vi "Test Counter Driven Output.vi"(8 "error in":errorcluster, 10 "TestCase in":refnum<class "Scan Engine Scripting API Modules.lvclass">, 11 "module test in":refnum<class "Module Test.lvclass">) -> (0 "error out":errorcluster, 2 "TestCase out":refnum<class "Scan Engine Scripting API Modules.lvclass">, 3 "module test out":refnum<class "Module Test.lvclass">)   [LabVIEW 2017, in "Module Test.lvclass"]
uses:
  Module Test.lvclass
  Scan Engine Scripting API Modules.lvclass
  C:/Program Files (x86)/National Instruments/LabVIEW 2017/vi.lib/addons/_JKI Toolkits/VI Tester/TestCase.llb/TestCase.lvclass
  Scripting/Modules/Mode Classes/Controls/counter driven output channel settings.ctl
  Scripting/Modules/Channel Classes/Counter Driven Output Channel/Counter Driven State.ctl
  Scripting/Modules/Mode Classes/Counter Driven Output Mode/Drive from Slot.ctl
  Module Test.lvclass/Module Test.ctl
  Scripting/Modules/Channel Classes/Counter Driven Output Channel/Counter Driven Output Channel.lvclass
  Scripting/Scan Engine Scripting.lvlib
  Scripting/Modules/Mode Classes/Counter Driven Output Mode/Counter Driven Output Mode.lvclass
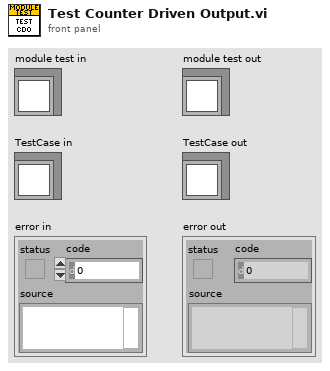
[diagram p1: front panel]
types:
  T1 = typedef "Scan Engine Scripting.lvlib/Counter Driven Output Mode.lvclass/Drive from Slot.ctl" = enum16{"Slot 1", "Slot 2", "Slot 3", "Slot 4", "Slot 5", "Slot 6", "Slot 7", "Slot 8"}
  T2 = typedef "Scan Engine Scripting.lvlib/counter driven output channel settings.ctl" = cluster{"name":string, "default value":bool, "counter driven state":T3}
  T3 = typedef "Scan Engine Scripting.lvlib/Counter Driven Output Channel.lvclass/Counter Driven State.ctl" = enum16{"Disabled", "Enabled"}
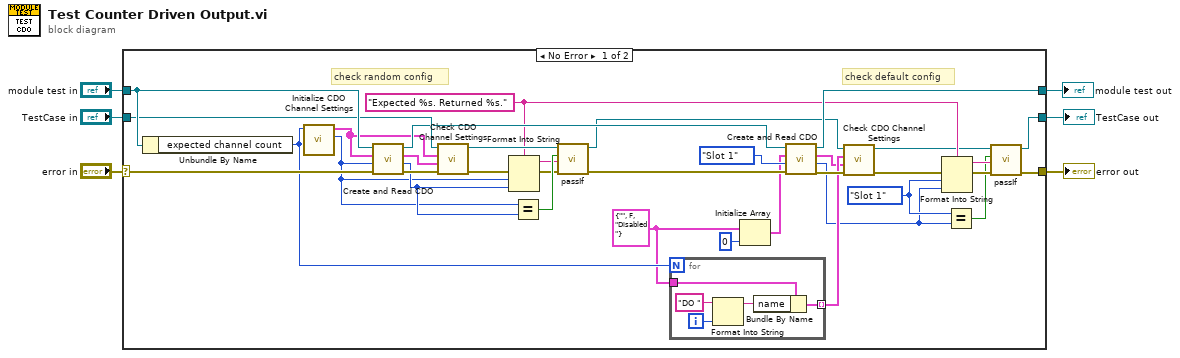
[diagram p0: block diagram]
diagram:
  n1 = case shown="No Error" "error in" {
    selector: "error in" -> [w41 w49]
    tunnel: [w24 w49] -> w5
    tunnel: [w30 w48] -> w3
    tunnel: "module test in" -> [w40 w48]
    tunnel: "TestCase in" -> [w38 w47]
    tunnel: [w25 w47] -> w1
    frame No Error {
      w23 = Drive_from_Slot."Slot 1" ("drive from slot")
      w15 = T2 {"name"="", "default value"=FALSE, "counter driven state"=enum."Disabled"} ("channel settings in")
      w26 = "Expected %s. Returned %s." ("format string")
      # "check default config"
      # "check random config"
      n2 = Unbundle By Name(w40) -> ("expected channel count"=w17:i32)
      n3 = call "Initialize CDO Channel Settings.vi"("array size"=w17) -> ("drive from slot"=w9:T1, "channel settings"=w7:T2[])  [unwired: 9 in]
      n4 = call-dynamic "Create and Read CDO.vi"("error in"=w41, "drive from slot in"=w9, "channel settings in"=w7, "Module Test in"=w40) -> ("error out"=w39:errorcluster, "drive from slot out"=w10:T1, "channel settings out"=w8:T2[], "Module Test out"=w31:refnum<class "Module Test.lvclass">)  [unwired: 4 in]
      n5 = call "Check CDO Channel Settings.vi"("error in"=w39, "read channel settings"=w8, "initial channel settings"=w7, "TestCase in"=w38) -> ("error out"=w34:errorcluster, "TestCase out"=w35:refnum<class "Scan Engine Scripting API Modules.lvclass">)  [unwired: 6 in]
      n6 = Format Into String(format string=w26, error in=w34, w9, w10) -> (resulting string=w33:string, error out=w36:errorcluster)  [unwired: 1 in]
      n7 = Equal?(x=w9, y=w10) -> (x = y?=w37:bool)
      n8 = call-dynamic "passIf.vi"("error in (no error)"=w36, "message (\"\")"=w33, "pass"=w37, "TestCase in"=w35) -> ("error out"=w32:errorcluster, "TestCase out"=w22:refnum<class "Scan Engine Scripting API Modules.lvclass">)  [unwired: 6 in]
      n9 = for {
        N: w17 -> [_]
        tunnel: [w43] -> w18 mode=indexing
        tunnel: w15 -> [w42]
        i -> [w46]
        n10 = Format Into String(initial string="DO ", w46) -> (resulting string=w44:string)  [unwired: 2 in, 1 out]
        n11 = Bundle By Name(cluster=w42, "name"=w44) -> (w43:T2)
      }
      n12 = Initialize Array(w15, 0 ("dimension size")) -> (w13:T2[])
      n13 = call-dynamic "Create and Read CDO.vi"("error in"=w32, "drive from slot in"=Drive_from_Slot."Slot 1", "channel settings in"=w13, "Module Test in"=w31) -> ("error out"=w20:errorcluster, "drive from slot out"=w12:T1, "channel settings out"=w11:T2[], "Module Test out"=w30:refnum<class "Module Test.lvclass">)  [unwired: 4 in]
      n14 = call "Check CDO Channel Settings.vi"("error in"=w20, "read channel settings"=w11, "initial channel settings"=w18, "TestCase in"=w22) -> ("error out"=w19:errorcluster, "TestCase out"=w21:refnum<class "Scan Engine Scripting API Modules.lvclass">)  [unwired: 6 in]
      n15 = Format Into String(format string=w26, error in=w19, w23, w12) -> (resulting string=w29:string, error out=w28:errorcluster)  [unwired: 1 in]
      n16 = Equal?(x=w23, y=w12) -> (x = y?=w27:bool)
      n17 = call-dynamic "passIf.vi"("error in (no error)"=w28, "message (\"\")"=w29, "pass"=w27, "TestCase in"=w21) -> ("error out"=w24:errorcluster, "TestCase out"=w25:refnum<class "Scan Engine Scripting API Modules.lvclass">)  [unwired: 6 in]
    }
    frame Error {
    }
  }
  "error out" <- w5
  "module test out" <- w3
  "TestCase out" <- w1
